vi "Set Post Processors.vi"(8 "error in (no error)":errorcluster, 10 "Post processors":string[](array[string]), 11 "Monitor-Pulse in":refnum<class "Monitor-Pulse.lvclass">) -> (0 "error out":errorcluster, 3 "Monitor-Pulse out":refnum<class "Monitor-Pulse.lvclass">)   [LabVIEW 2015, in "Monitor-Pulse.lvclass"]
uses:
  Monitor-Pulse.lvclass
  <vilib>/ActorFramework/Message Enqueuer/Message Enqueuer.lvclass/Message Enqueuer.ctl
  <vilib>/ActorFramework/Message Enqueuer/Enqueue.vi
  <vilib>/ActorFramework/Message Priority Queue/Priority Enqueue.vi
  Measure_core/Measure Object Messages/Time to subscribe Msg/Time to subscribe Msg.lvclass
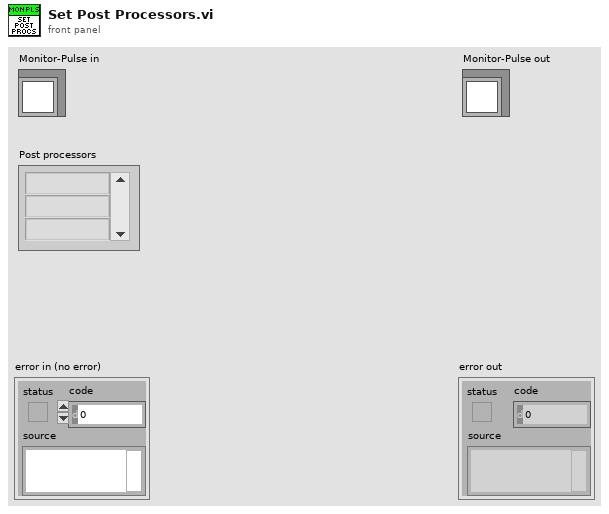
[diagram p1: front panel]
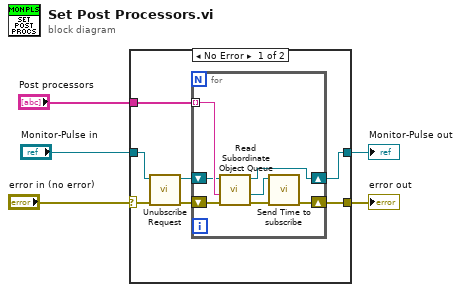
[diagram p0: block diagram]
diagram:
  n1 = case shown="No Error" "error in (no error)" {
    selector: "error in (no error)" -> [w10 w21]
    tunnel: [w9 w21] -> w4
    tunnel: [w7 w20] -> w2
    tunnel: "Monitor-Pulse in" -> [w8 w20]
    tunnel: "Post processors" -> [w6 _]
    frame No Error {
      n2 = call-dynamic "Unubscribe Request.vi"("error in (no error)"=w10, "Measure Object in"=w8) -> ("error out"=w11:errorcluster, "Measure Object out"=w12:refnum<class "Monitor-Pulse.lvclass">)  [unwired: 8 in]
      n3 = for {
        tunnel: w6 -> [w19] mode=indexing
        shift-right: [w13] -> w7
        shift-left: w12 -> [w18]
        shift-right: [w14] -> w9
        shift-left: w11 -> [w17]
        n4 = call-dynamic "Read Subordinate Object Queue.vi"("error in (no error)"=w17, "Name"=w19, "Measure Object in"=w18) -> ("error out"=w15:errorcluster, "Object Enqueuer"=w16:refnum<class "Message Enqueuer.lvclass">, "Measure Object out"=w13:refnum<class "Monitor-Pulse.lvclass">)  [unwired: 5 in, 1 out]
        n5 = call "Send Time to subscribe.vi"("error in (no error)"=w15, "Message Enqueuer"=w16) -> ("error out"=w14:errorcluster)  [unwired: 8 in, 1 out]
      }
    }
    frame Error {
    }
  }
  "error out" <- w4
  "Monitor-Pulse out" <- w2
